vi "runrate1.vi"() -> ()   [LabVIEW 2012]
uses:
  <vilib>/addons/database/Auxilliary.llb/DB Tools Cursor Type.ctl
  <vilib>/addons/database/Connection.llb/DB Tools Open Connec (Path).vi
  <vilib>/addons/database/Connection.llb/Conn Execute.vi
  <vilib>/addons/database/Recordset.llb/Rec Fetch Recordset Data (R).vi
  <vilib>/addons/database/Recordset.llb/Rec Destroy - Connection.vi
  <vilib>/addons/database/_DB Variant To Data/Database Variant To Data.xnode
  <vilib>/addons/database/NI_Database_API.lvlib
panel:
  in  "Machine":string
  in  "EndDate":string="2014/11/23"
  in  "BegDate":string="2014/11/01"
  out "Table Control":string[][](table)
  out "transposed array":string[][](array[string])
  out "array":string[][](array[string])
  out "recordset data":variant[][](array[variant])
  out "error out":errorcluster
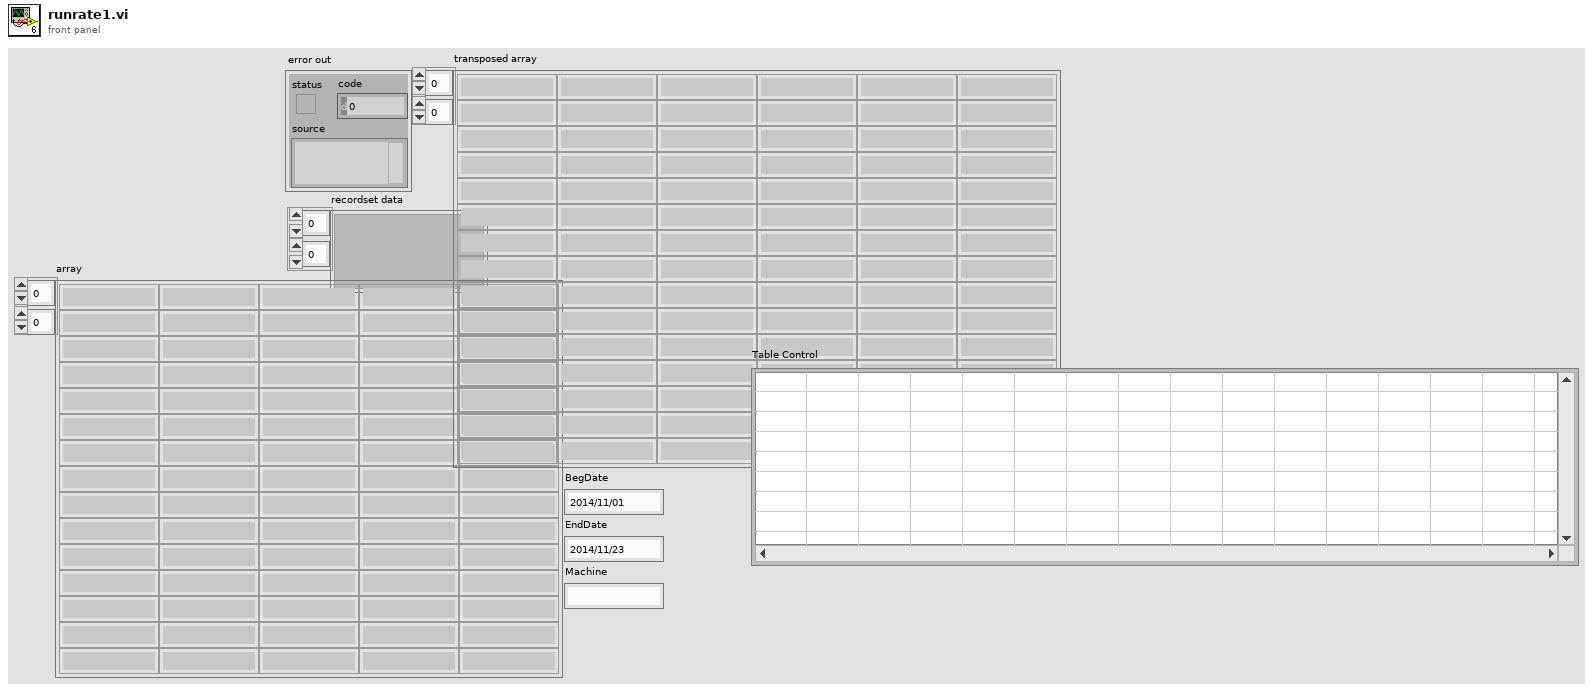
[diagram p1: front panel]
types:
  T1 = typedef "NI_Database_API.lvlib/DB Tools Cursor Type.ctl" = enum16{"forward-only", "keyset", "dynamic", "static"}
  T2 = typedef "NI_Database_API.lvlib/Conn ObjectReference.ctl" = refnum<k1>
  T3 = typedef "NI_Database_API.lvlib/Rec ObjectReference.ctl" = refnum<k1>
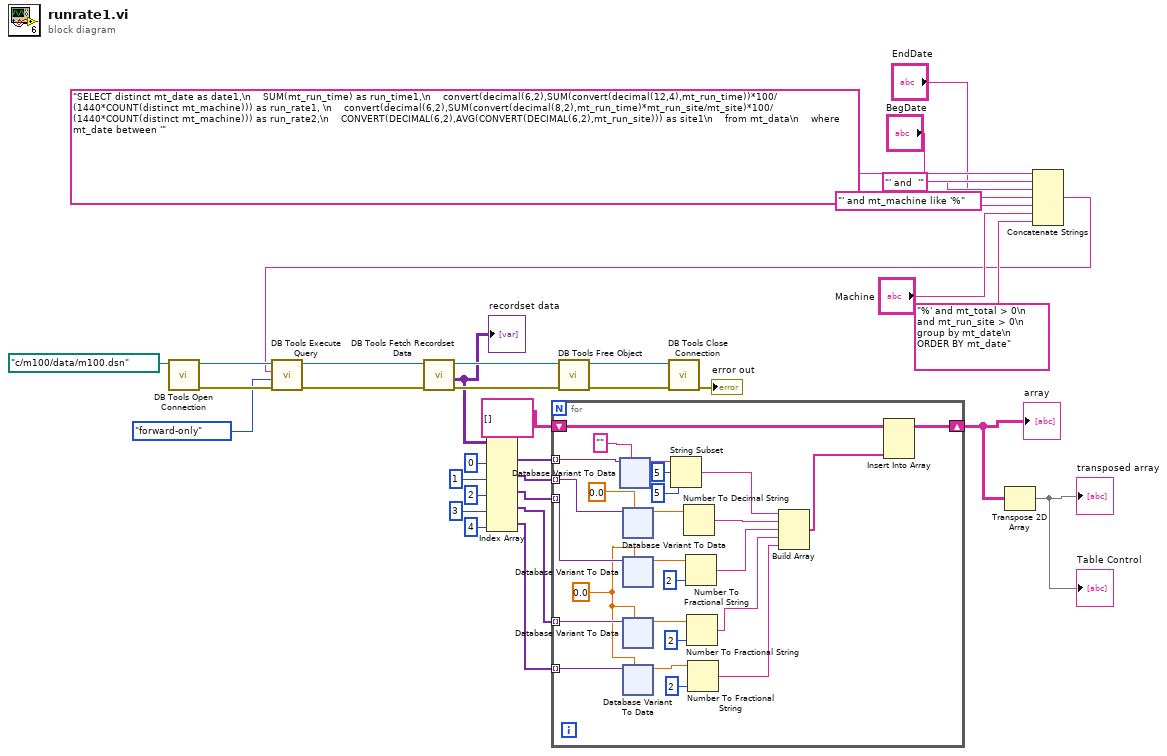
[diagram p0: block diagram]
diagram:
  n1 = call-poly <vilib>:"DB Tools Open Connection.vi"("connection information"=path "c:/m100/data/m100.dsn") -> ("error out"=w29:errorcluster, "connection reference"=w33:T2)  [unwired: 7 in]
  n2 = Concatenate Strings("SELECT distinct mt_date as date1,\n    SUM(mt_run_time) as run_time1,\n    convert(decimal(6,2),SUM(convert(decimal(12,4),mt_run_time))*100/(1440*COUNT(distinct mt_machine))) as run_rate1, \n    convert(decimal(6,2),SUM(convert(decimal(8,2),mt_run_time)*mt_run_site/mt_site)*100/(1440*COUNT(distinct mt_machine))) as run_rate2,\n    CONVERT(DECIMAL(6,2),AVG(CONVERT(DECIMAL(6,2),mt_run_site))) as site1\n    from mt_data\n    where mt_date between '" ("SQL query"), "BegDate", "' and  '" ("string"), "EndDate", "' and mt_machine like '%" ("string"), "Machine", "%' and mt_total > 0\n      and mt_run_site > 0\n     group by mt_date\n     ORDER BY mt_date" ("string")) -> (w1:string)
  n3 = call-poly <vilib>:"DB Tools Execute Query.vi"("error in (no error)"=w29, "cursor type"=DB_Tools_Cursor_Type."forward-only", "SQL query"=w1, "connection reference"=w33) -> ("error out"=w28:errorcluster, "recordset reference"=w32:T3)  [unwired: 4 in]
  n4 = call-poly <vilib>:"DB Tools Fetch Recordset Data.vi"("error in (no error)"=w28, "recordset reference"=w32) -> ("error out"=w27:errorcluster, "recordset data"=w22:variant[][], "recordset reference out"=w31:T3)  [unwired: 3 in]
  "recordset data" <- w22
  n5 = Index Array(array=w22, index (col) #1=0 ("disabled index (col)"), index (col) #2=1 ("index (col)"), index (col) #3=2 ("index (col)"), index (col) #4=3 ("index (col)"), index (col) #5=4 ("index (col)")) -> (element #1=w17:variant[], element #2=w16:variant[], element #3=w15:variant[], element #4=w13:variant[], element #5=w12:variant[])  [unwired: 5 in]
  n6 = for {
    tunnel: w17 -> [w59] mode=indexing
    tunnel: w16 -> [w57] mode=indexing
    tunnel: w15 -> [w56] mode=indexing
    tunnel: w13 -> [w55] mode=indexing
    tunnel: w12 -> [w54] mode=indexing
    shift-right: [w43] -> w10
    shift-left: string[][] [] ("array") -> [w42]
    w41 = 0.0
    n7 = xnode "Database Variant To Data"("database variant"=w59, "type"="") -> ("data"=w37:string)  [unwired: 1 in, 1 out]
    n8 = xnode "Database Variant To Data"("database variant"=w57, "type"=0.0) -> ("data"=w49:dbl)  [unwired: 1 in, 1 out]
    n9 = xnode "Database Variant To Data"("database variant"=w56, "type"=w41) -> ("data"=w50:dbl)  [unwired: 1 in, 1 out]
    n10 = xnode "Database Variant To Data"("database variant"=w55, "type"=w41) -> ("data"=w51:dbl)  [unwired: 1 in, 1 out]
    n11 = xnode "Database Variant To Data"("database variant"=w54, "type"=w41) -> ("data"=w52:dbl)  [unwired: 1 in, 1 out]
    n12 = String Subset(string=w37, offset (0)=5, length (rest)=5 ("length (rest)")) -> (substring=w36:string)
    n13 = Number To Decimal String(number=w49) -> (decimal integer string=w48:string)  [unwired: 1 in]
    n14 = Number To Fractional String(number=w50, precision (6)=i16 2) -> (F-format string=w47:string)  [unwired: 2 in]
    n15 = Number To Fractional String(number=w51, precision (6)=i16 2) -> (F-format string=w46:string)  [unwired: 2 in]
    n16 = Number To Fractional String(number=w52, precision (6)=i16 2) -> (F-format string=w45:string)  [unwired: 2 in]
    n17 = Build Array(w36, w48, w47, w46, w45) -> (w44:string[])
    n18 = Insert Into Array(array=w42, new element=w44) -> (w43:string[][])  [unwired: 2 in]
  }
  "array" <- w10
  n19 = call-poly <vilib>:"DB Tools Free Object.vi"("error in (no error)"=w27, "recordset reference"=w31) -> ("error out"=w26:errorcluster, "connection reference"=w30:T2)  [unwired: 8 in]
  n20 = call <vilib>:"DB Tools Close Connection.vi"("error in (no error)"=w26, "connection reference"=w30) -> ("error out"=→"error out":errorcluster)  [unwired: 5 in]
  n21 = Transpose 2D Array(2D array=w10) -> (transposed array=→"transposed array" →"Table Control":string[][])
